vi "RM.Globals.vi"() -> ()   [LabVIEW 2016, in "FPGA Resource Manager.lvlib"]
uses:
  FPGA Resource Manager.lvlib
panel:
  in  "Tab Control":enum32{"Shared", "Server", "Client"}(tab)=enum."Server"
  in  "String":string
  in  "RM.SERVER.GUID":string="RM.SERVER.GUID"
  in  "RM.SERVER.DATABASE":string="RM.SERVER.DATABASE"
  in  "RM.CLIENT.GUID":string="RM.CLIENT.GUID"
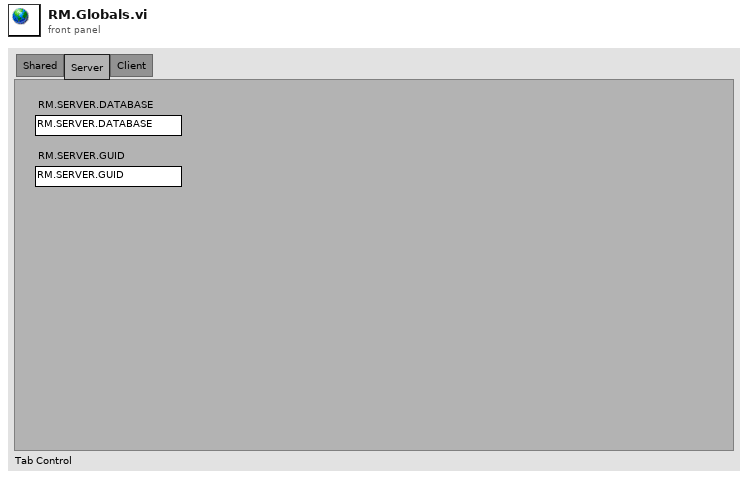
[diagram p1: front panel]
diagram:
